vi "L0_DelayLine_File_Appender_NU.vi"(0 "Vin":dbl, 1 "CH":dbl, 2 "DelayLine":dbl, 3 "Status":dbl=63.0, 4 "Path":dbl, 5 "Vmeas":dbl format="%#_6f", 6 "Measured Delay":dbl format="%#_6f", 7 "file path (dialog if empty)":path) -> (19 "appended array":dbl[](array[numeric]), 27 "file path (dialog if empty) 2":path)   [LabVIEW 2012]
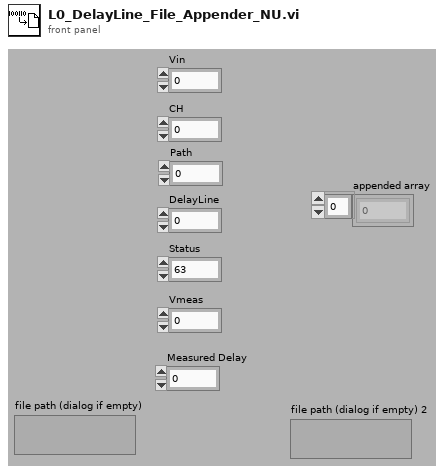
[diagram p1: front panel]
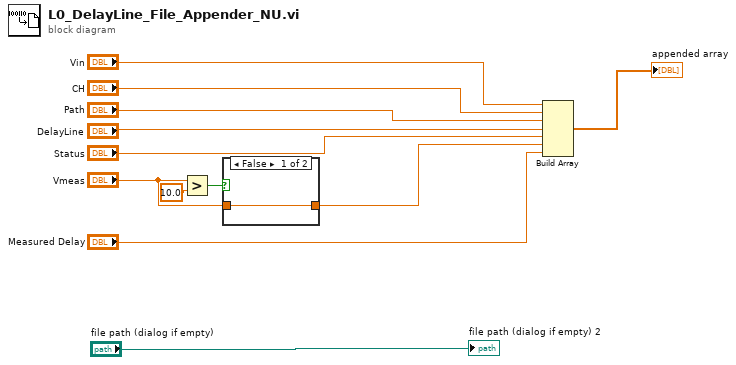
[diagram p0: block diagram]
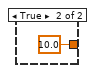
[diagram p2: hidden frame]
diagram:
  n1 = Greater?(x="Vmeas", y=10.0) -> (0:w7:bool)
  n2 = case shown="False" w7 {
    tunnel: "Vmeas" -> [w13 _]
    tunnel: [w13 10.0 ("Vmeas")] -> w5
    frame False {
    }
    frame True {
    }
  }
  n3 = Build Array("Vin", "CH", "Path", "DelayLine", "Status", w5, "Measured Delay") -> (→"appended array":dbl[])
  "file path (dialog if empty) 2" <- "file path (dialog if empty)"
